vi "ReadWrite.ProcessData.Read.vi"(7 "Ignore Reset Values?":bool=TRUE, 8 "error in (no error)":errorcluster, 10 "timeout ms":i32=100, 11 "ReadWrite in":refnum<class "ReadWrite.lvclass">) -> (0 "error out":errorcluster, 1 "Timeout?":bool, 2 "Values":dbl[](array[numeric]), 3 "ReadWrite out":refnum<class "ReadWrite.lvclass">, 5 "Detect?":bool[](array[boolean]))   [LabVIEW 2027, in "Data Access Engine.lvlib" / "ReadWrite.lvclass"]
uses:
  ReadWrite.lvclass
  ReadWrite.lvclass/ReadWrite.ctl
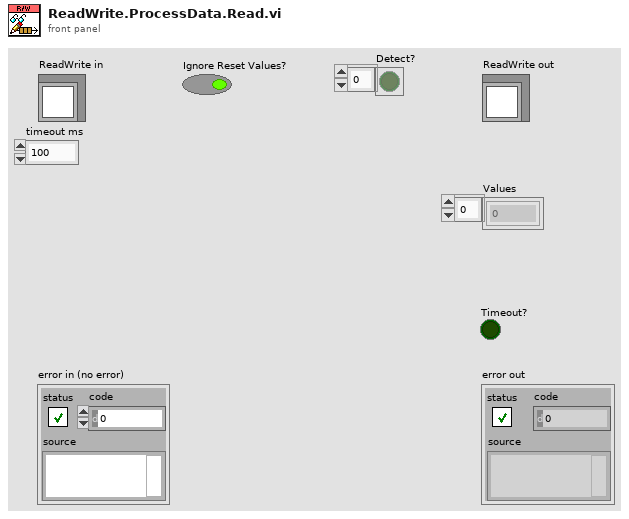
[diagram p1: front panel]
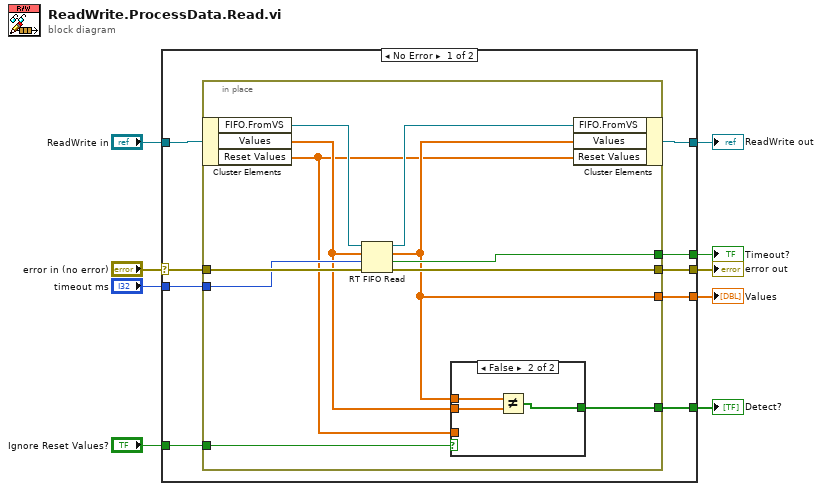
[diagram p0: block diagram]
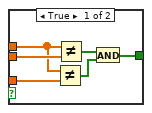
[diagram p2: hidden frame]
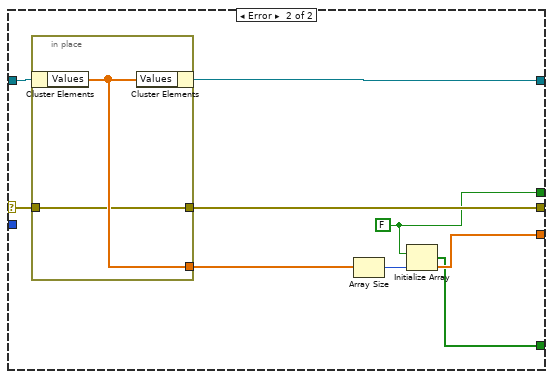
[diagram p3: hidden frame]
diagram:
  n1 = case shown="No Error" "error in (no error)" {
    selector: "error in (no error)" -> [w18 w43]
    tunnel: [w17 w44] -> w8
    tunnel: [w14 w45] -> w6
    tunnel: "ReadWrite in" -> [w15 w46]
    tunnel: [w16 w41] -> w5
    tunnel: "timeout ms" -> [w13 _]
    tunnel: [w12 w39] -> w3
    tunnel: [w11 w40] -> w2
    tunnel: "Ignore Reset Values?" -> [w10 _]
    frame No Error {
      n2 = in-place {
        in-place-border: w18 -> [w28]
        in-place-border: [w22] -> w17
        in-place-border: [w21] -> w16
        in-place-border: w13 -> [w26]
        in-place-border: [w25] -> w12
        in-place-border: [w23] -> w11
        in-place-border: w10 -> [w20]
        n3 = in-place-cluster #1(w15) -> ("FIFO.FromVS"=w29:refnum<k33>, "Values"=w24:dbl[], "Reset Values"=w19:dbl[])
        n4 = RT FIFO Read(0:w29, 1:w24, 2:w26, 3:w28) -> (8:w27:refnum<k33>, 9:w21:dbl[], 10:w25:bool, 11:w22:errorcluster)  [unwired: 1 out]
        n5 = case shown="False" w20 {
          tunnel: w24 -> [w35 w38]
          tunnel: [w31 w36] -> w23
          tunnel: w21 -> [w33 w37]
          tunnel: w19 -> [w32 _]
          frame True {
            n6 = Not Equal?(x=w33, y=w32) -> (x != y?=w30:bool[])
            n7 = Not Equal?(x=w33, y=w35) -> (x != y?=w34:bool[])
            n8 = And(x=w34, y=w30) -> (x .and. y?=w31:bool[])
          }
          frame False {
            n9 = Not Equal?(x=w37, y=w38) -> (x != y?=w36:bool[])
          }
        }
        n10 = in-place-cluster #1("FIFO.FromVS"=w27, "Values"=w21, "Reset Values"=w19) -> (w14:refnum<class "ReadWrite.lvclass">)
      }
    }
    frame Error {
      w39 = FALSE ("empty?")
      n11 = in-place {
        in-place-border: [w48] -> w41
        in-place-border: [w47] -> w44
        in-place-border: w43 -> [w47]
        n12 = in-place-cluster #2(w46) -> ("Values"=w48:dbl[])
        n13 = in-place-cluster #2("Values"=w48) -> (w45:refnum<class "ReadWrite.lvclass">)
      }
      n14 = Array Size(array=w41) -> (size(s)=w42:i32)
      n15 = Initialize Array(w39, w42) -> (w40:bool[])
    }
  }
  "error out" <- w8
  "ReadWrite out" <- w6
  "Values" <- w5
  "Timeout?" <- w3
  "Detect?" <- w2
